vi "I32NonDim_to_umNonDim.vi"(6 "-10 to 10V range?":bool, 8 "Max Value [um]":dbl, 11 "Input":i16=5000) -> (2 "x*y":dbl)   [LabVIEW 2023]
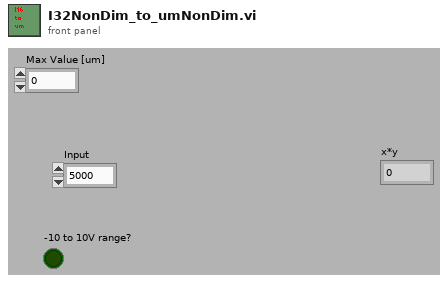
[diagram p1: front panel]
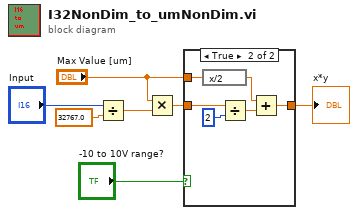
[diagram p0: block diagram]
diagram:
  n1 = Divide(x="Input", y=32767.0 ("n")) -> (x/y=w5:dbl)
  n2 = Multiply(x="Max Value [um]", y=w5) -> (x*y=w2:dbl)
  n3 = case shown="True" "-10 to 10V range?" {
    tunnel: w2 -> [w8 w13]
    tunnel: [w8 w9] -> w4
    tunnel: "Max Value [um]" -> [_ w11]
    frame False {
    }
    frame True {
      n4 = expression code="x/2"(w11) -> (w10:dbl)
      n5 = Divide(x=w13, y=2) -> (x/y=w12:dbl)
      n6 = Add(x=w10, y=w12) -> (x+y=w9:dbl)
    }
  }
  "x*y" <- w4
